vi "Configure_Burst.vi"(6 "Impedancia":enum16{"50", "600", "HiZ"}(ring), 7 "# ciclos":i32, 8 "error in (no error)":errorcluster, 9 "Frequency (Hz)":dbl=10.0, 10 "Amplitude (Vrms)":dbl=5.0, 11 "VISA resource name":refnum<visa-resource-name>) -> (0 "error out":errorcluster, 3 "VISA resource name out":refnum<visa-resource-name>)   [LabVIEW 2019, in "DS360.lvlib"]
uses:
  DS360.lvlib
panel:
  out "resulting string":string
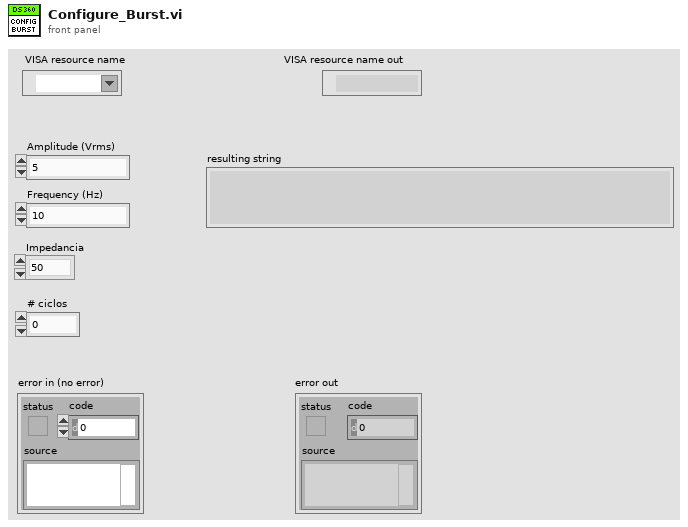
[diagram p1: front panel]
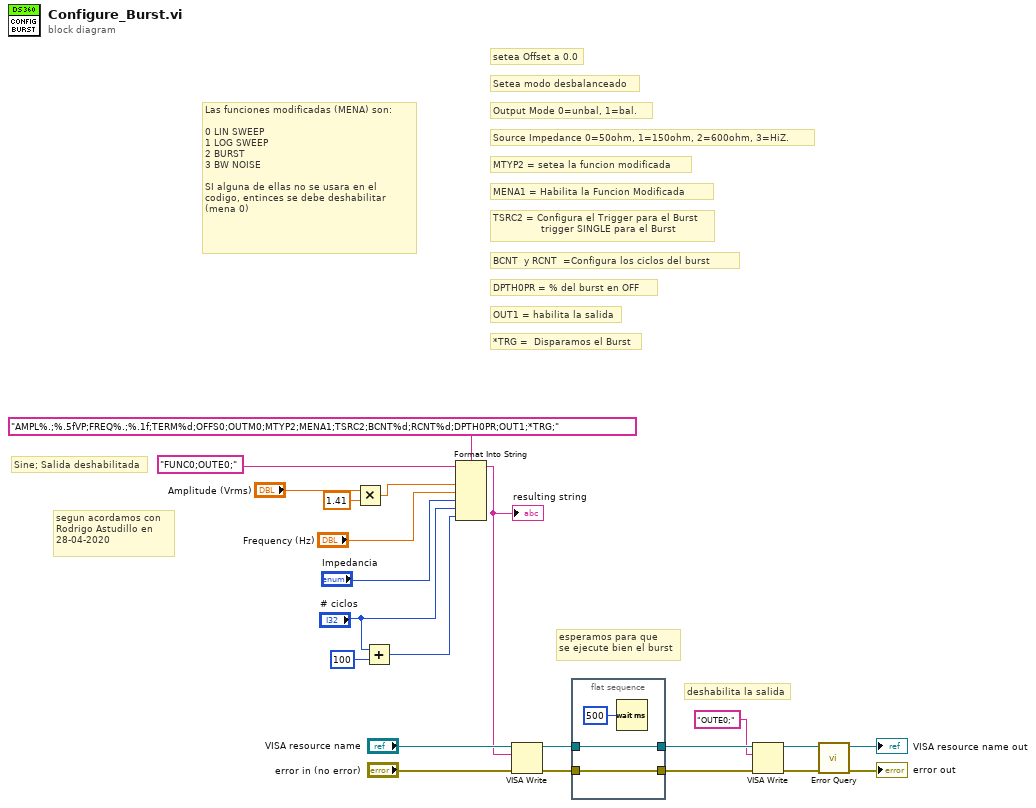
[diagram p0: block diagram]
diagram:
  # "deshabilita la salida"
  # "esperamos para que\nse ejecute bien el burst"
  # "*TRG =  Disparamos el Burst"
  # "OUT1 = habilita la salida"
  # "DPTH0PR = % del burst en OFF"
  # "BCNT  y RCNT  =Configura los ciclos del burst"
  # "TSRC2 = Configura el Trigger para el Burst\n                trigger SINGLE para el Burst"
  # "MENA1 = Habilita la Funcion Modificada"
  # "MTYP2 = setea la funcion modificada"
  # "Source Impedance 0=50ohm, 1=150ohm, 2=600ohm, 3=HiZ."
  # "Output Mode 0=unbal, 1=bal."
  # "Setea modo desbalanceado"
  # "setea Offset a 0.0"
  # "Las funciones modificadas (MENA) son:\n\n0 LIN SWEEP\n1 LOG SWEEP\n2 BURST\n3 BW NOISE\n\nSI alguna de ellas no se usara en el\ncodigo, entinces se debe deshabilitar\n(mena 0)"
  # "segun acordamos con\nRodrigo Astudillo en\n28-04-2020"
  # "Sine; Salida deshabilitada"
  n1 = Multiply(x="Amplitude (Vrms)", y=1.41) -> (x*y=w13:dbl)
  n2 = Add(x="# ciclos", y=100) -> (x+y=w8:i32)
  n3 = Format Into String(format string="AMPL%.;%.5fVP;FREQ%.;%.1f;TERM%d;OFFS0;OUTM0;MTYP2;MENA1;TSRC2;BCNT%d;RCNT%d;DPTH0PR;OUT1;*TRG;", initial string="FUNC0;OUTE0;" ("string (\"\")"), w13, "Frequency (Hz)", "Impedancia", "# ciclos", w8) -> (resulting string=w11:string)  [unwired: 1 in, 1 out]
  "resulting string" <- w11
  n4 = VISA Write(VISA resource name="VISA resource name", write buffer=w11, error in (no error)="error in (no error)") -> (VISA resource name out=w6:refnum<visa-resource-name>, error out=w7:errorcluster)  [unwired: 1 out]
  n5 = flat-sequence {
    tunnel: w7 -> [w24]
    tunnel: [w24] -> w3
    tunnel: w6 -> [w23]
    tunnel: [w23] -> w2
    frame #0 {
      n6 = Wait (ms)(milliseconds to wait=u32 500) -> ()  [unwired: 1 out]
    }
  }
  n7 = VISA Write(VISA resource name=w2, write buffer="OUTE0;" ("string (\"\")"), error in (no error)=w3) -> (VISA resource name out=w5:refnum<visa-resource-name>, error out=w4:errorcluster)  [unwired: 1 out]
  n8 = call "Error Query.vi"("error in (no error)"=w4, "VISA resource name"=w5) -> ("error out"=→"error out":errorcluster, "VISA resource name out"=→"VISA resource name out":refnum<visa-resource-name>)  [unwired: 6 in, 2 out]
